vi "Read Self-Test Result Code.vi"(8 "error in (no error)":errorcluster, 11 "CS++DeviceGUIActor in":refnum<class "CS++DeviceGUIActor.lvclass">) -> (0 "error out":errorcluster, 2 "Self-Test Result Code":i32, 3 "CS++DeviceGUIActor out":refnum<class "CS++DeviceGUIActor.lvclass">)   [LabVIEW 2015, in "CS++DeviceGUIActor.lvlib" / "CS++DeviceGUIActor.lvclass"]
doc: "This parameter contains the value returned from the instrument self test. Zero means success. For any other code, see the instrument's operation manual.\n\nThis value has been read at launch time of actor once."
uses:
  CS++DeviceGUIActor.lvclass
  CS++DeviceGUIActor.lvclass/CS++DeviceGUIActor.ctl
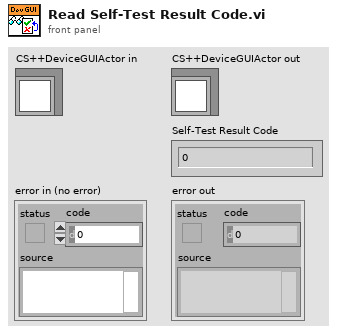
[diagram p1: front panel]
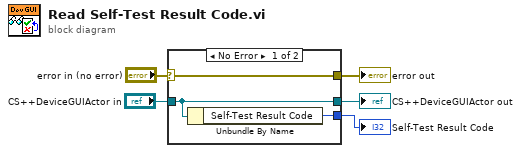
[diagram p0: block diagram]
diagram:
  n1 = case shown="No Error" "error in (no error)" {
    selector: "error in (no error)" -> [w8 w9]
    tunnel: [w8 w9] -> w4
    tunnel: [w7 w10] -> w2
    tunnel: "CS++DeviceGUIActor in" -> [w7 w10]
    tunnel: [w6 _] -> w1
    frame No Error {
      n2 = Unbundle By Name(w7) -> ("Self-Test Result Code"=w6:i32)
    }
    frame Error {
    }
  }
  "error out" <- w4
  "CS++DeviceGUIActor out" <- w2
  "Self-Test Result Code" <- w1
